vi "PAN_StartCom.vi"(8 "error in (no error)":errorcluster, 9 "configfile":path, 10 "Front Panel Window:Open":bool, 11 "coms to run":path[](array[path])) -> (2 "info":string)   [LabVIEW 2016]
panel:
  out "error out":errorcluster
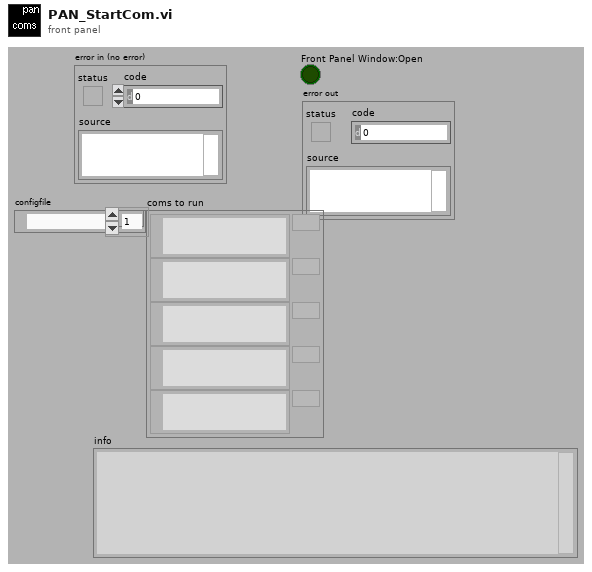
[diagram p1: front panel]
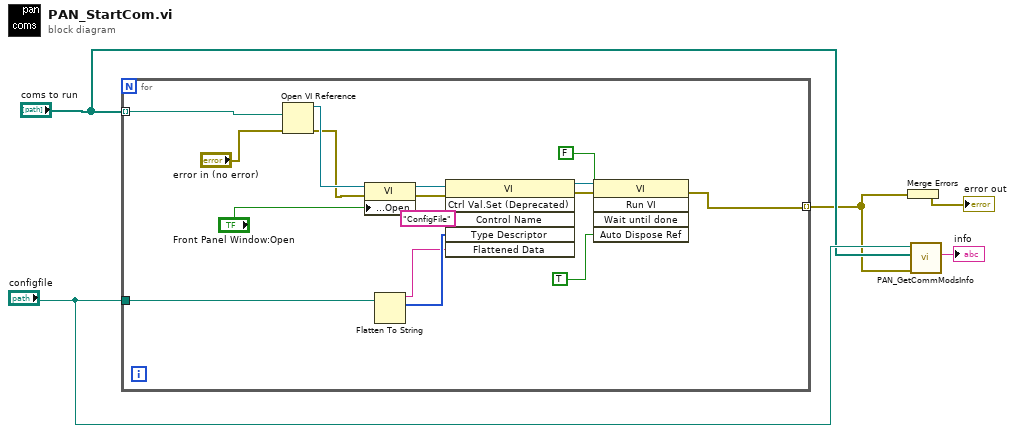
[diagram p0: block diagram]
diagram:
  n1 = for {
    tunnel: "coms to run" -> [w9] mode=indexing
    tunnel: "configfile" -> [w8]
    tunnel: [w6] -> w1 mode=indexing
    n2 = Open VI Reference(vi path=w9, error in (no error)="error in (no error)") -> (vi reference=w12:refnum<vi>, error out=w10:errorcluster)  [unwired: 4 out]
    n3 = property class="VI"(reference=w12, error in=w10, "Front Panel.Open"="Front Panel Window:Open") -> (reference out=w20:refnum<vi>, error out=w14:errorcluster)
    n4 = Flatten To String(anything=w8) -> (data string=w15:string, type string=w16:i16[])  [unwired: 1 in, 3 out]
    n5 = invoke class="VI" method="Ctrl Val.Set (Deprecated)"(reference=w20, error in=w14, "Control Name"="ConfigFile", "Type Descriptor"=w16, "Flattened Data"=w15) -> (reference out=w19:refnum<vi>, error out=w13:errorcluster)  [unwired: 1 in, 4 out]
    n6 = invoke class="VI" method="Run VI"(reference=w19, error in=w13, "Wait until done"=FALSE ("Wait Until Done"), "Auto Dispose Ref"=TRUE ("Auto Dispose Reference")) -> (error out=w6:errorcluster)  [unwired: 1 in, 4 out]
  }
  n7 = Merge Errors(w1) -> (→"error out":errorcluster)
  n8 = call "PAN_GetCommModsInfo.vi"("errors"=w1, "coms to run"="coms to run", "configfile"="configfile") -> ("info"=→"info":string)  [unwired: 8 out]
